vi "optionsAcq_getAll.vi"(0 "reference":refnum<class "OSA.lvclass">, 7 "error in (no error)":errorcluster) -> (8 "gain/offset auto":bool, 9 "gain out":u16, 10 "attenuator auto":bool, 11 "attenuator":bool, 12 "airMesure out":T5, 13 "intervall out (ms)":u32, 14 "apodisation":T4, 15 "smoothing specrtum":T2, 16 "rolling out":bool, 17 "zeroFill out":u8, 18 "offset read":i32, 19 "gain_relative":dbl, 20 "duplicate reference":refnum<class "OSA.lvclass">, 21 "average out":u32, 23 "cycleCounting out":bool, 24 "smoothing interferogram":T2, 25 "phaseCorrection":T3, 26 "PD sensitivity mode out":T1, 27 "error out":errorcluster)   [LabVIEW 2010, in "OSA.lvclass"]
uses:
  OSA.lvclass
  typeDef/airMeasure.ctl
  typeDef/apodisation.ctl
  _misc/Thorlabs_FTS_misc.llb/interferogram_smoothing.ctl
  typeDef/phaseCorrection.ctl
  _misc/Thorlabs_FTS_misc.llb/PDTemperatureMode.ctl
  OSA20X_misc.lvlib
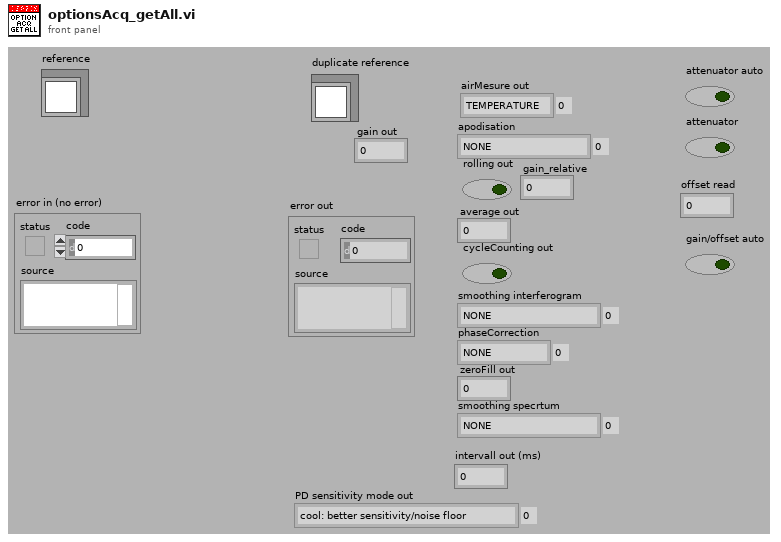
[diagram p1: front panel]
types:
  T1 = typedef "OSA20X_misc.lvlib/PDTemperatureMode.ctl" = enum16{"cool: better sensitivity/noise floor", "warm: extended wl range"}
  T2 = typedef "OSA20X_misc.lvlib/interferogram_smoothing.ctl" = enum16{"NONE", "BINOMIAL", "SAVITSKY_GOLAY", "FOURIER", "MOVING_AVERAGE", "GAUSSIAN"}
  T3 = typedef "OSA.lvclass/phaseCorrection.ctl" = enum16{"NONE", "MERTZ", "FORMAN", "MERTZ_FILE", "FORMAN_FILE", "FUTURE COMP."}
  T4 = typedef "OSA.lvclass/apodisation.ctl" = enum16{"NONE", "NORTON_BEER_WEAK", "NORTON_BEER_MEDIUM", "NORTON_BEER_STRONG", "TRIANGULAR", "COSINE", "HANN", "HAMMING", "BLACKMANHARRIS3", "BLACKMANHARRIS4", "GAUSSIAN"}
  T5 = typedef "OSA.lvclass/airMeasure.ctl" = enum16{"TEMPERATURE", "PRESSURE"}
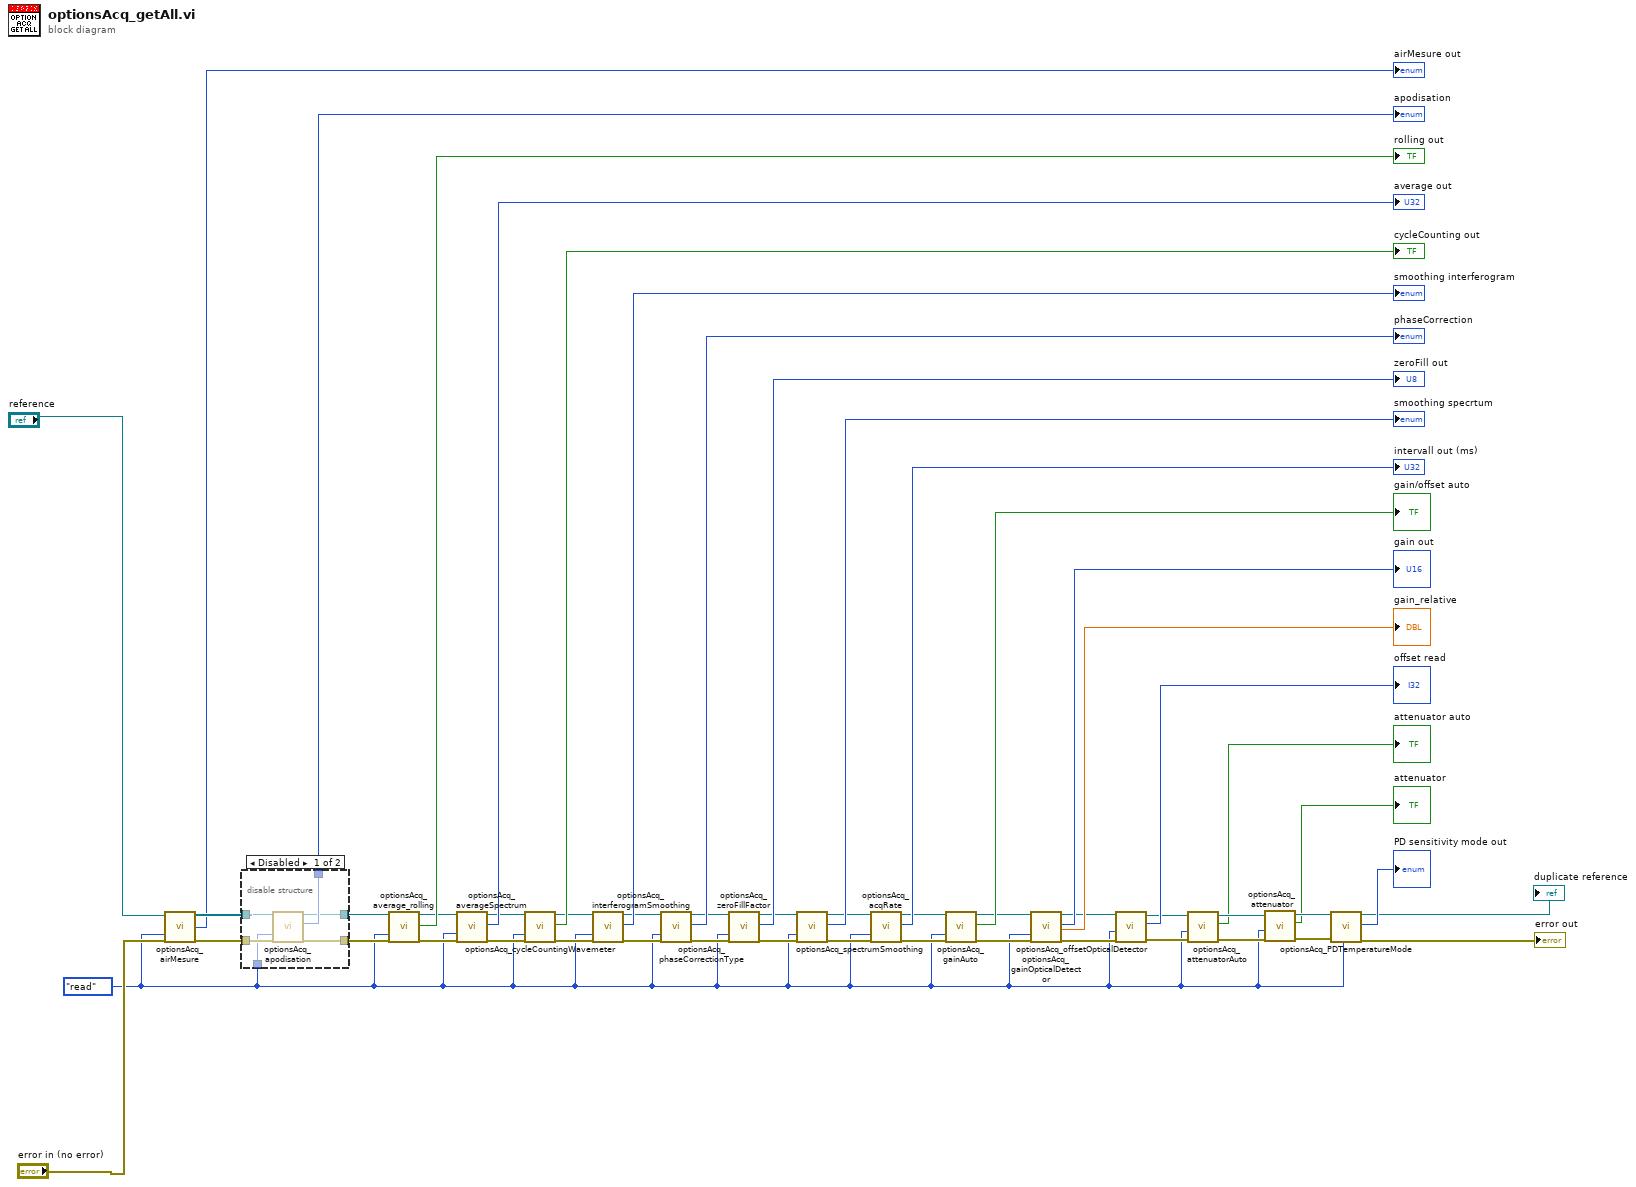
[diagram p0: block diagram]
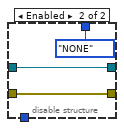
[diagram p2: hidden frame]
diagram:
  w3 = enum16{"read", "write"}."read" ("readWrite")
  n1 = call "optionsAcq_airMesure.vi"("reference"="reference", "readWrite"=w3, "error in (no error)"="error in (no error)") -> ("duplicate reference"=w41:refnum<class "OSA.lvclass">, "airMesure out"=→"airMesure out":T5, "error out"=w33:errorcluster)  [unwired: 13 in, 1 out]
  n2 = disable-structure shown="Disabled" {
    disable-tunnel: [w58 apodisation."NONE" ("apodisation")] -> w49
    disable-tunnel: w41 -> [w57 w61]
    disable-tunnel: [w56 w61] -> w40
    disable-tunnel: w33 -> [w55 w60]
    disable-tunnel: [w54 w60] -> w32
    disable-tunnel: w3 -> [w53 _]
    frame Disabled {
      n3 = call "optionsAcq_apodisation.vi"("reference"=w57, "readWrite"=w53, "error in (no error)"=w55) -> ("duplicate reference"=w56:refnum<class "OSA.lvclass">, "apodisation"=w58:T4, "error out"=w54:errorcluster)  [unwired: 13 in, 1 out]
    }
    frame Enabled {
    }
  }
  "apodisation" <- w49
  n4 = call "optionsAcq_average_rolling.vi"("reference"=w40, "readWrite"=w3, "error in (no error)"=w32) -> ("duplicate reference"=w39:refnum<class "OSA.lvclass">, "rolling out"=→"rolling out":bool, "error out"=w31:errorcluster)  [unwired: 13 in, 1 out]
  n5 = call "optionsAcq_averageSpectrum.vi"("reference"=w39, "readWrite"=w3, "error in (no error)"=w31) -> ("duplicate reference"=w38:refnum<class "OSA.lvclass">, "average out"=→"average out":u32, "error out"=w30:errorcluster)  [unwired: 13 in, 1 out]
  n6 = call-dynamic "optionsAcq_cycleCountingWavemeter.vi"("reference"=w38, "readWrite"=w3, "error in (no error)"=w30) -> ("duplicate reference"=w37:refnum<class "OSA.lvclass">, "cycleCounting out"=→"cycleCounting out":bool, "error out"=w29:errorcluster)  [unwired: 13 in, 1 out]
  n7 = call-dynamic "optionsAcq_interferogramSmoothing.vi"("reference"=w37, "readWrite"=w3, "error in (no error)"=w29) -> ("duplicate reference"=w36:refnum<class "OSA.lvclass">, "smoothing out"=→"smoothing interferogram":T2, "error out"=w28:errorcluster)  [unwired: 11 in, 3 out]
  n8 = call "optionsAcq_phaseCorrectionType.vi"("reference"=w36, "readWrite"=w3, "error in (no error)"=w28) -> ("duplicate reference"=w35:refnum<class "OSA.lvclass">, "phaseCorrection"=→"phaseCorrection":T3, "error out"=w27:errorcluster)  [unwired: 13 in, 1 out]
  n9 = call "optionsAcq_zeroFillFactor.vi"("reference"=w35, "readWrite"=w3, "error in (no error)"=w27) -> ("duplicate reference"=w34:refnum<class "OSA.lvclass">, "zeroFill out"=→"zeroFill out":u8, "error out"=w26:errorcluster)  [unwired: 13 in, 1 out]
  n10 = call-dynamic "optionsAcq_spectrumSmoothing.vi"("reference"=w34, "readWrite"=w3, "error in (no error)"=w26) -> ("duplicate reference"=w24:refnum<class "OSA.lvclass">, "smoothing out"=→"smoothing specrtum":T2, "error out"=w25:errorcluster)  [unwired: 11 in, 3 out]
  n11 = call "optionsAcq_acqRate.vi"("reference"=w24, "readWrite"=w3, "error in (no error)"=w25) -> ("duplicate reference"=w21:refnum<class "OSA.lvclass">, "intervall out (ms)"=→"intervall out (ms)":u32, "error out"=w22:errorcluster)  [unwired: 14 in]
  n12 = call-dynamic "optionsAcq_gainAuto.vi"("reference"=w21, "readWrite"=w3, "error in (no error)"=w22) -> ("duplicate reference"=w19:refnum<class "OSA.lvclass">, "auto out"=→"gain/offset auto":bool, "error out"=w18:errorcluster)  [unwired: 13 in, 1 out]
  n13 = call-dynamic "optionsAcq_gainOpticalDetector.vi"("reference"=w19, "readWrite"=w3, "error in (no error)"=w18) -> ("duplicate reference"=w11:refnum<class "OSA.lvclass">, "gain_idx  out"=→"gain out":u16, "gain_relative"=→"gain_relative":dbl, "error out"=w12:errorcluster)  [unwired: 12 in, 1 out]
  n14 = call-dynamic "optionsAcq_offsetOpticalDetector.vi"("error in (no error)"=w12, "readWrite"=w3, "Thorlabs_OSA_64 in"=w11) -> ("error out"=w8:errorcluster, "offset read"=→"offset read":i32, "Thorlabs_OSA_64 out"=w9:refnum<class "OSA.lvclass">)  [unwired: 5 in, 1 out]
  n15 = call-dynamic "optionsAcq_attenuatorAuto.vi"("error in (no error)"=w8, "readWrite"=w3, "Thorlabs_OSA_64 in"=w9) -> ("error out"=w7:errorcluster, "auto out"=→"attenuator auto":bool, "Thorlabs_OSA_64 out"=w6:refnum<class "OSA.lvclass">)  [unwired: 5 in, 1 out]
  n16 = call-dynamic "optionsAcq_attenuator.vi"("error in (no error)"=w7, "readWrite"=w3, "Thorlabs_OSA_64 in"=w6) -> ("error out"=w4:errorcluster, "attenuator out"=→"attenuator":bool, "Thorlabs_OSA_64 out"=w5:refnum<class "OSA.lvclass">)  [unwired: 4 in, 2 out]
  n17 = call-dynamic "optionsAcq_PDTemperatureMode.vi"("reference"=w5, "error in (no error)"=w4, "read/write"=w3) -> ("duplicate reference"=→"duplicate reference":refnum<class "OSA.lvclass">, "PD sensitivity mode out"=→"PD sensitivity mode out":T1, "error out"=→"error out":errorcluster)  [unwired: 13 in, 1 out]
